vi "picture.clear.vi"(7 "Keep Keyboard? (T)":bool=TRUE, 8 "error in":errorcluster, 11 "midi-ui in":refnum<class "midi-ui.lvclass">) -> (0 "error out":errorcluster, 3 "midi-ui out":refnum<class "midi-ui.lvclass">)   [LabVIEW 2020, in "midi-ui.lvclass"]
uses:
  midi-ui.lvclass
  midi-ui.lvclass/midi-ui.ctl
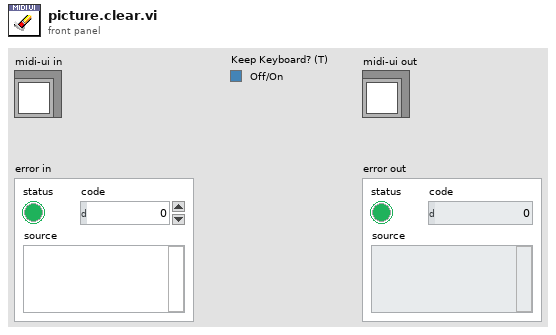
[diagram p1: front panel]
types:
  T1 = typedef "midi-ui.lvclass/privatedata.ctl" = cluster{"White Key Length":dbl, "White Key Width":dbl, "Black Key Length":dbl, "Polygon Corners by Name":map{string, cluster{"x":dbl, "y":dbl}[]}, "Anticlockwise rotations [0-3] (0)":i32, "Polygon Corners by Note Name":map{string, cluster{"x":dbl, "y":dbl}[]}, "Picture Control":refnum<vi>, "Owning VI":refnum<vi>, "Control Index":i32, "Note Bounds by Note Name":map{string, cluster{"max":dbl, "min":dbl}}, "Notes on screen":cluster{"Note Value":enum8{"C-2", "C#-2", "D-2", "D#-2", "E-2", "F-2", "F#-2", "G-2", "G#-2", "A-2", "A#-2", "B-2", "C-1", "C#-1", "D-1", "D#-1", "E-1", "F-1", "F#-1", "G-1", "G#-1", "A-1", "A#-1", "B-1", "C0", "C#0", "D0", "D#0", "E0", "F0", "F#0", "G0", "G#0", "A0", "A#0", "B0", "C1", "C#1", "D1", "D#1", "E1", "F1", "F#1", "G1", "G#1", "A1", "A#1", "B1", "C2", "C#2", "D2", "D#2", "E2", "F2", "F#2", "G2", "G#2", "A2", "A#2", "B2", "C3", "C#3", "D3", "D#3", "E3", "F3", "F#3", "G3", "G#3", "A3", "A#3", "B3", "C4", "C#4", "D4", "D#4", "E4", "F4", "F#4", "G4", "G#4", "A4", "A#4", "B4", "C5", "C#5", "D5", "D#5", "E5", "F5", "F#5", "G5", "G#5", "A5", "A#5", "B5", "C6", "C#6", "D6", "D#6", "E6", "F6", "F#6", "G6", "G#6", "A6", "A#6", "B6", "C7", "C#7", "D7", "D#7", "E7", "F7", "F#7", "G7", "G#7", "A7", "A#7", "B7", "C8", "C#8", "D8", "D#8", "E8", "F8", "F#8", "G"}, "End Time":u32, "Start Time":u32}[], "Polygon Pictures by Note Name":map{i32, cluster{"Note On":picture, "Note Off":picture}}, "keyboard":picture[], "Keyboard Note Index by Name":map{i32, i32}, "music":picture[]}
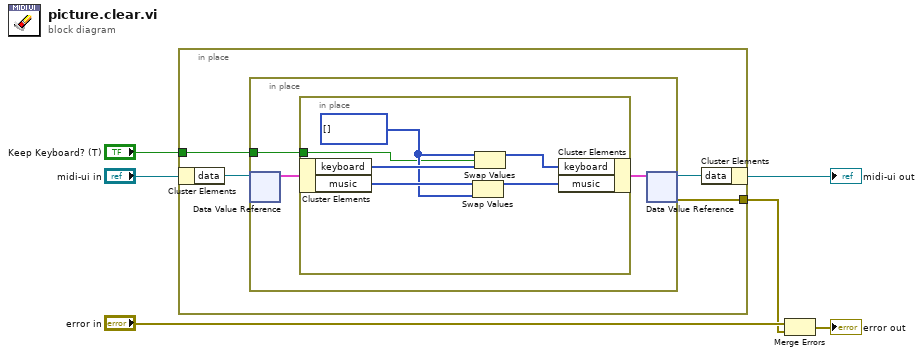
[diagram p0: block diagram]
diagram:
  n1 = in-place {
    in-place-border: "Keep Keyboard? (T)" -> [w8]
    in-place-border: [w7] -> w2
    n2 = in-place-cluster #1("midi-ui in") -> ("data"=w10:refnum<data-value>)
    n3 = in-place {
      in-place-border: w8 -> [w11]
      n4 = in-place-dvr #2(w10) -> (w13:T1)  [unwired: 1 out]
      n5 = in-place {
        in-place-border: w11 -> [w14]
        w16 = picture[] []
        n6 = in-place-cluster #3(w13) -> ("keyboard"=w19:picture[], "music"=w17:picture[])
        n7 = Swap Values(12:w17, 14:w16) -> (1:w15:picture[])  [unwired: 1 in, 1 out]
        n8 = Swap Values(12:w16, 13:w14, 14:w19) -> (1:w18:picture[])  [unwired: 1 out]
        n9 = in-place-cluster #3("keyboard"=w18, "music"=w15) -> (w12:T1)
      }
      n10 = in-place-dvr #2(w12) -> (w9:refnum<data-value>, w7:errorcluster)
    }
    n11 = in-place-cluster #1("data"=w9) -> (→"midi-ui out":refnum<class "midi-ui.lvclass">)
  }
  n12 = Merge Errors("error in", w2) -> (→"error out":errorcluster)
